vi "HomeUarm.vi"(8 "error in":errorcluster, 11 "Machine In":refnum<visa-resource-name>) -> (0 "error out":errorcluster, 3 "Machine Out":refnum<visa-resource-name>)   [LabVIEW 2017]
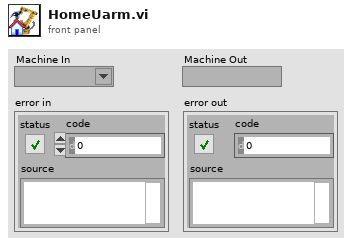
[diagram p1: front panel]
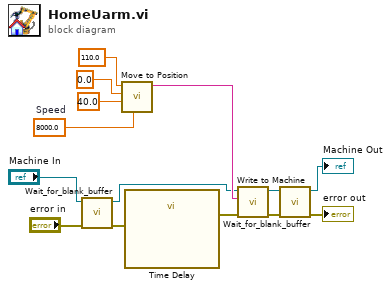
[diagram p0: block diagram]
diagram:
  w12 = 8000.0  # Speed
  n1 = call "Wait_for_blank_buffer.vi"("error in (no error)"="error in", "VISA Refnum in"="Machine In") -> ("error out"=w2:errorcluster, "VISA Refnum out"=w7:refnum<visa-resource-name>)  [unwired: 8 in]
  n2 = call "Move to Position.vi"("Speed"=w12, "Z-Position"=40.0, "Y-Position"=0.0, "X-Position"=110.0) -> ("G-Code String"=w8:string)  [unwired: 7 in]
  n3 = call "Time Delay"("error in (no error)"=w2) -> ("error out"=w1:errorcluster)  [unwired: 10 in]
  n4 = call "Write to Machine .vi"("error in (no error)"=w1, "G-Code String In"=w8, "Machine In"=w7) -> ("error out"=w6:errorcluster, "Machine Out"=w5:refnum<visa-resource-name>)  [unwired: 7 in]
  n5 = call "Wait_for_blank_buffer.vi"("error in (no error)"=w6, "VISA Refnum in"=w5) -> ("error out"=→"error out":errorcluster, "VISA Refnum out"=→"Machine Out":refnum<visa-resource-name>)  [unwired: 8 in]
